vi "Close_Test.vi"(8 "error in (no error)":errorcluster caption="entrée d'erreur (pas d'erreur)", 11 "Test_With_Inst en entrée":refnum<class "Test_With_Inst.lvclass">) -> (0 "error out":errorcluster caption="sortie d'erreur", 3 "Test_With_Inst en sortie":refnum<class "Test_With_Inst.lvclass">)   [LabVIEW 2020, in "Library Test.lvlib" / "Test_With_Inst.lvclass"]
uses:
  Test_With_Inst.lvclass
  C:/Users/ngarcin/OneDrive - Altyor/Standard TB/Class/Test/Test (Default)/Test (Default).lvclass
  Test (Default)/Test (Default).lvclass
  Instrument/Instrument (Default)/Class Instrument (Default).lvclass
  Test_With_Inst.lvclass/Test_With_Inst.ctl
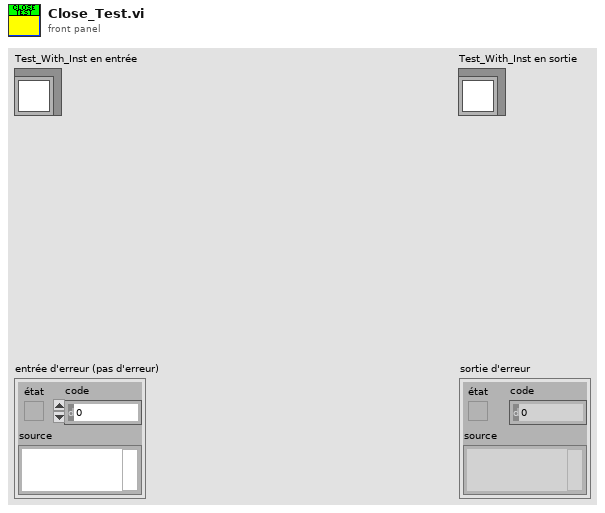
[diagram p1: front panel]
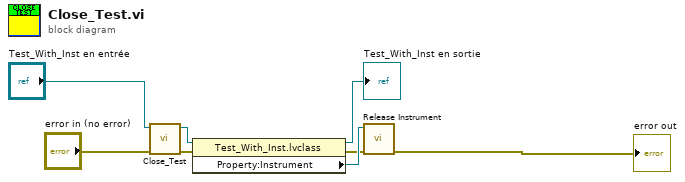
[diagram p0: block diagram]
diagram:
  n1 = call-parent "Close_Test.vi"("error in (no error)"="error in (no error)", "Test (Default) en entrée"="Test_With_Inst en entrée") -> ("error out"=w2:errorcluster, "Test (Default) en sortie"=w6:refnum<class "Test_With_Inst.lvclass">)  [unwired: 8 in]
  n2 = property class="Test_With_Inst.lvclass"(reference=w6, error in=w2) -> (reference out=→"Test_With_Inst en sortie":refnum<class "Test_With_Inst.lvclass">, error out=w4:errorcluster, "Property:Instrument"=w5:refnum<class "Class Instrument (Default).lvclass">)
  n3 = call-dynamic "Release Instrument.vi"("error in (no error)"=w4, "Class Instrument (Default) en entrée"=w5) -> ("error out"=→"error out":errorcluster)  [unwired: 8 in, 1 out]
